vi "Read Active Logs.vi"(8 "error in (no error)":errorcluster, 11 "ActiveModulesContainer in":refnum<class "ActiveModulesContainer.lvclass">) -> (0 "error out":errorcluster, 2 "Logs":T1, 3 "ActiveModulesContainer out":refnum<class "ActiveModulesContainer.lvclass">)   [LabVIEW 2019, in "ActiveModulesContainer.lvlib" / "ActiveModulesContainer.lvclass"]
uses:
  ActiveModulesContainer.lvclass
  <vilib>/ActorFramework/Message Enqueuer/Message Enqueuer.lvclass
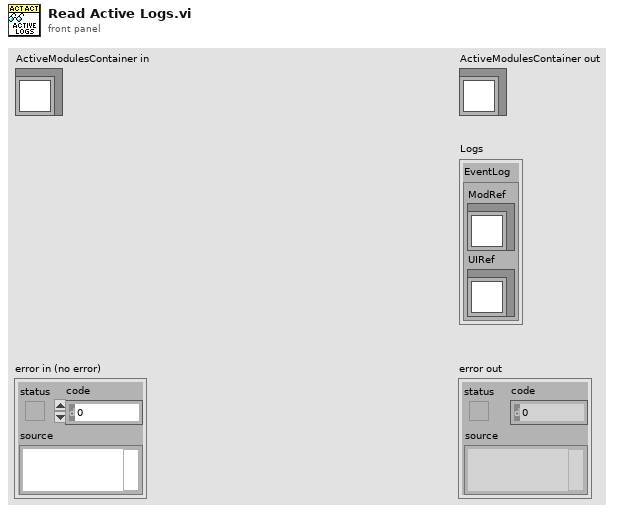
[diagram p1: front panel]
types:
  T1 = cluster{"EventLog":cluster{"ModRef":refnum<class "Message Enqueuer.lvclass">, "UIRef":refnum<class "Message Enqueuer.lvclass">}}
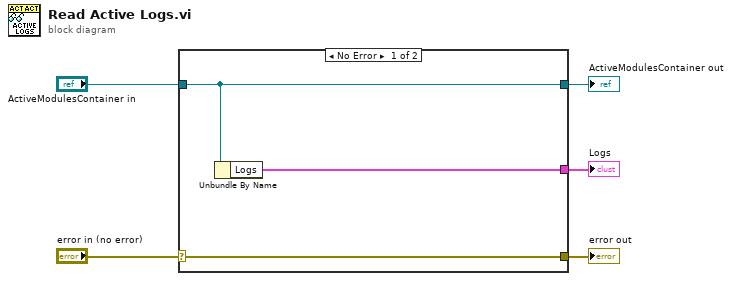
[diagram p0: block diagram]
diagram:
  n1 = case shown="No Error" "error in (no error)" {
    selector: "error in (no error)" -> [w8 w9]
    tunnel: [w8 w9] -> w4
    tunnel: [w7 w10] -> w2
    tunnel: "ActiveModulesContainer in" -> [w7 w10]
    tunnel: [w6 _] -> w1
    frame No Error {
      n2 = Unbundle By Name(w7) -> ("Logs"=w6:T1)
    }
    frame Error {
    }
  }
  "error out" <- w4
  "ActiveModulesContainer out" <- w2
  "Logs" <- w1
